vi "проба_ASK.vi"() -> ()   [LabVIEW 2017]
uses:
  <vilib>/addons/Modulation/Analog/support/mod_Set Error Source.vi
  <vilib>/addons/Modulation/Digital/Support/Common/Validators/mod_AWGN Validate.vi
  <vilib>/addons/Modulation/Digital/Impairments/subVIs/mod_createSeeds.vi
  <vilib>/addons/Modulation/Digital/Support/Common/Validators/mod_Validate Samples Per Symbol.vi
  <vilib>/addons/Modulation/Analog/support/Validators/mod_Validate Complex Waveform.vi
  <vilib>/addons/Modulation/Analog/support/Validators/mod_WFErrorHandler.vi
  <vilib>/addons/Modulation/Digital/General/MT Generate ASK system parameters (M).vi
  <vilib>/addons/Modulation/Digital/Support/Common/Validators/mod_Generate Filter Coefficients Validate.vi
  <vilib>/addons/Modulation/Digital/General/subVIs/mod_Generate Filter Coefficients.vi
  <vilib>/addons/Modulation/Digital/General/subVIs/mod_Generate Bits PN Sequence.vi
  <vilib>/Analysis/1siggen.llb/Gaussian White Noise (obs 90).vi
  <vilib>/addons/Modulation/niDMT.lvlib
  <vilib>/addons/Modulation/Digital/General/MT Align to Ideal Symbols (Generic).vi
  <vilib>/addons/Modulation/Digital/Equalization/MT ASK Feedforward Equalizer (LMS) (Specify coefficients).vi
  <vilib>/addons/Modulation/Digital/Demodulation/MT Measure ASK Quadrature Impairments.vi
  <vilib>/addons/Modulation/Digital/Demodulation/MT Calculate BER After Trigger (PN Sequence).vi
  <vilib>/addons/Modulation/Digital/General/MT Apply Matched Filter (Generic).vi
panel:
  out "output bit stream":i8[](array[numeric])
  in  "pulse shaping filter (none)":T1(ring)
  in  "M-ASK (2)":i32=2
  in  "samples per symbol (16)":i32=16
  out "Массив без пауз":dbl[](array[numeric])
  out "Массив с паузами":dbl[](array[numeric])
  in  "Сколько битов брать":i32=4
  in  "Количество бит":i32=8
  out "Вырезка из массива":dbl[](array[numeric])
  out "Биты на выходе 1":dbl[](array[numeric])
  # "ASK Parameters"
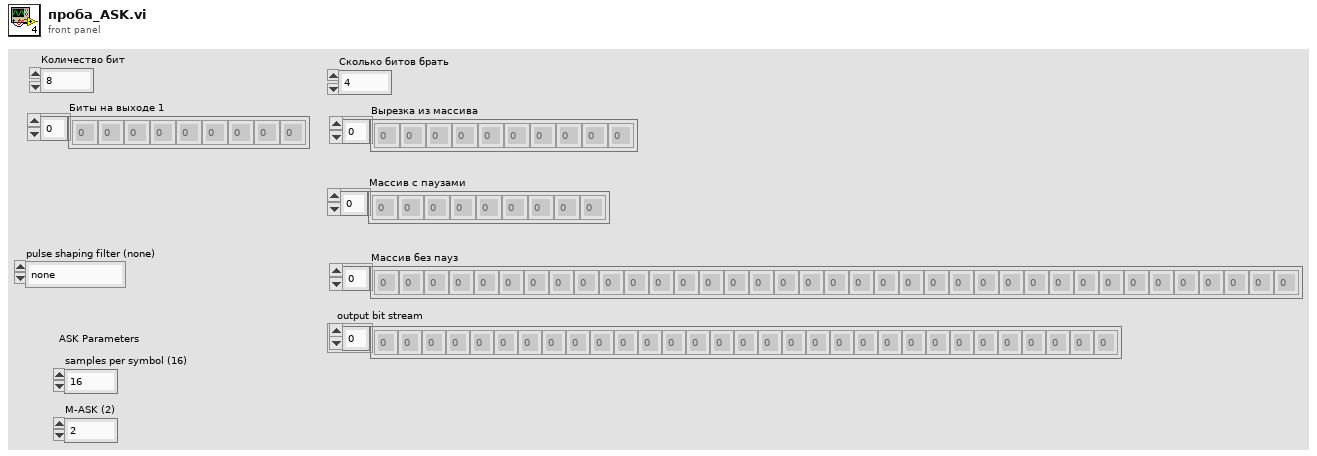
[diagram p1: front panel]
types:
  T1 = enum16{"none", "Raised Cosine", "Root Raised Cos", "Gaussian"}
  T2 = enum16{"FSK", "PSK", "QAM", "MSK", "PAM", "ASK", "CPM"}
  T3 = cluster{"samples per symbol (16)":i32, "symbol map":cdb[]}
  T4 = typedef "niAMT.lvlib/Complex Data Waveform.ctl" = cluster{"t0":dbl, "dt":dbl, "Y":cdb[]}
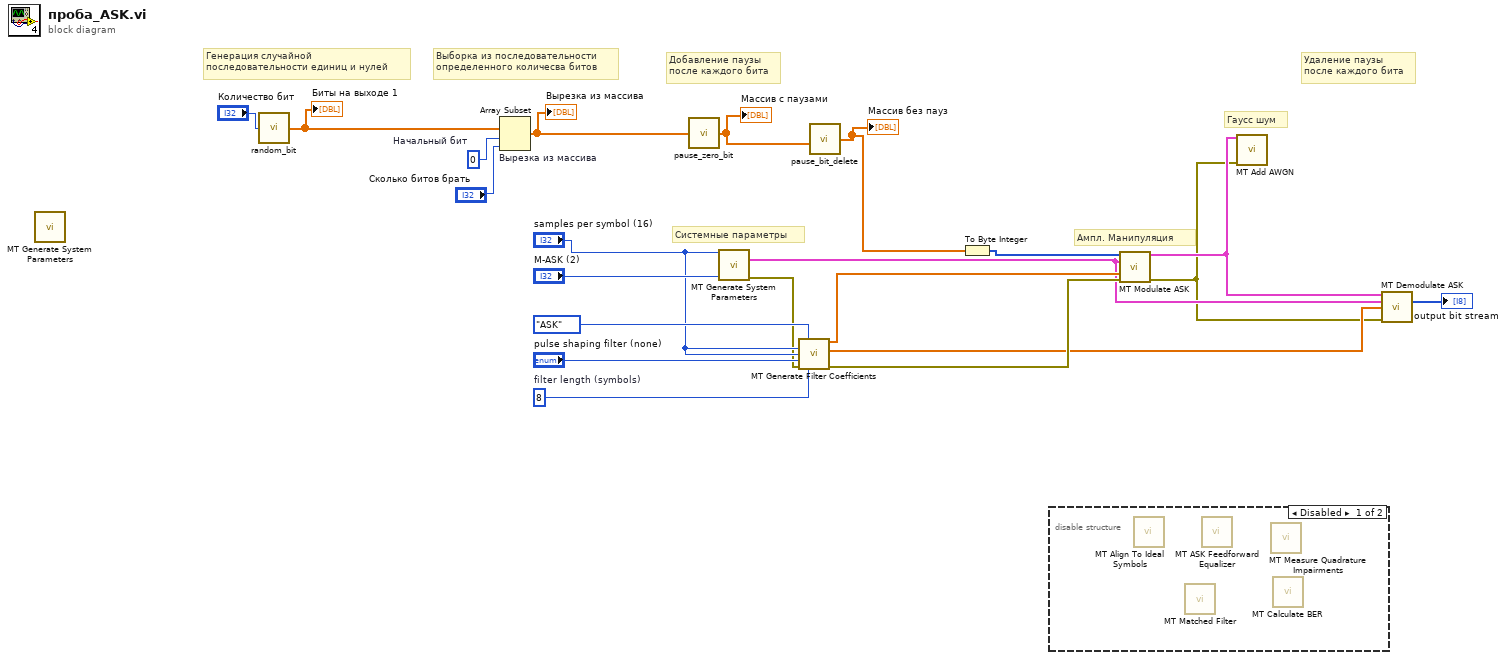
[diagram p0: block diagram]
diagram:
  w12 = 8  # filter length (symbols)
  w21 = 0  # Начальный бит
  # "Системные параметры"
  # "Ампл. Манипуляция"
  # "Гаусс шум"
  # "Удаление паузы \nпосле каждого бита"
  # "Добавление паузы \nпосле каждого бита"
  # "Выборка из последовательности\nопределенного количесва битов"
  # "Генерация случайной \nпоследовательности единиц и нулей"
  n1 = call-poly <vilib>:"MT Generate System Parameters.vi"() -> ()  [unwired: 3 in, 13 out]
  n2 = call "random_bit.vi"("Количество бит"="Количество бит") -> ("Биты на выходе 1"=w19:dbl[])
  "Биты на выходе 1" <- w19
  n3 = Array Subset "Вырезка из массива"(array=w19, index=w21, length="Сколько битов брать") -> (w17:dbl[])
  "Вырезка из массива" <- w17
  n4 = call "pause_zero_bit.vi"("Входная последовательность"=w17) -> ("Массив с паузами"=w3:dbl[])
  "Массив с паузами" <- w3
  n5 = call-poly <vilib>:"MT Generate System Parameters.vi"("samples per symbol (16)"="samples per symbol (16)", "M-ASK (2)"="M-ASK (2)") -> ("ASK system parameters"=w6:T3, "error out"=w10:errorcluster)  [unwired: 11 in, 1 out]
  n6 = call <vilib>:"MT Generate Filter Coefficients.vi"("pulse shaping filter (none)"="pulse shaping filter (none)", "modulation type"=T2."ASK", "pulse shaping samples per symbol (16)"="samples per symbol (16)", "matched samples per symbol (16)"="samples per symbol (16)", "error in (no error)"=w10, "filter length (symbols)"=w12) -> ("pulse shaping filter coefficients"=w11:dbl[], "matched filter coefficients"=w8:dbl[], "error out"=w9:errorcluster)  [unwired: 1 in, 6 out]
  n7 = call "pause_bit_delete.vi"("Массив с паузами"=w3) -> ("Массив без пауз"=w2:dbl[])
  "Массив без пауз" <- w2
  n8 = To Byte Integer(number=w2) -> (8bit integer=w1:i8[])
  n9 = disable-structure shown="Disabled" {
    frame Disabled {
      n10 = call-poly <vilib>:"MT Align To Ideal Symbols.vi"() -> ()  [unwired: 5 in, 11 out]
      n11 = call-poly <vilib>:"MT Matched Filter.vi"() -> ()  [unwired: 5 in, 11 out]
      n12 = call-poly <vilib>:"MT ASK Feedforward Equalizer.vi"() -> ()  [unwired: 7 in, 9 out]
      n13 = call-poly <vilib>:"MT Measure Quadrature Impairments.vi"() -> ()  [unwired: 6 in, 10 out]
      n14 = call-poly <vilib>:"MT Calculate BER.vi"() -> ()  [unwired: 6 in, 10 out]
    }
    frame Enabled {
    }
  }
  n15 = call <vilib>:"MT Modulate ASK.vi"("input bit stream"=w1, "ASK system parameters"=w6, "pulse shaping filter coefficients"=w11, "error in (no error)"=w9) -> ("output complex waveform"=w7:T4, "error out"=w5:errorcluster)  [unwired: 3 in, 7 out]
  n16 = call <vilib>:"MT Add AWGN.vi"("input complex waveform"=w7, "error in (no error)"=w5) -> ()  [unwired: 5 in, 9 out]
  n17 = call <vilib>:"MT Demodulate ASK.vi"("input complex waveform"=w7, "ASK system parameters"=w6, "matched filter coefficients"=w8, "error in (no error)"=w5) -> ("output bit stream"=→"output bit stream":i8[])  [unwired: 7 in, 4 out]
